vi "HEWH RLT PRAT.vi"() -> ()   [LabVIEW 2016] (continued)
        n823 = call "HEWH Gather Test Data.vi"("MW100"=w1875, "Core HEWH Data Station A"=w1870, "GEA2?"="GEA2_A?", "Yokogawa WT210"=w1863, "error in (no error)"=w1876, "Laurel IP Address"=w1853, "Draw Count"=w1852, "Use Emerson 5700?"=w1847) -> ("Core HEWH Data Station A"=w1854:T12, "MW100 Full Data"=w1868:string[][], "error out"=w1869:errorcluster)  [unwired: 6 in, 3 out]
        n824 = Unbundle By Name(w1854) -> ("LV Program"=w1860:T24)
        n825 = local read "Draw Station"() -> (w1864:string)
        n826 = call "HEWH RLT Selected MW100 TCs.vi"("Collect Power Data"="DAQ for A", "Show Flow Data"="Show Stand Override Flow Data A", "Station ID"=w1851, "Current Drawing Station"=w1864, "Error In"=w1869, "Station A Channels, MW100"=w1866, "MW100 Full Data"=w1868, "LV Program"=w1860) -> ("Error Out"=w1862:errorcluster, "TC Data"=w1857:string[][], "RMS Current (Amps)"=w1865:dbl, "Data (Label,Data)"=w1867:string[][])
        n827 = Build Array (concatenate)(w1880, w1867) -> (w1879:string[][])
        n828 = local read "Test CompleteA"() -> (w1848:bool)
        n829 = call "HEWH Tank Display.vi"("TC Data"=w1857, "LV Program"=w1860, "Min Temp (°F)"=50.0, "Max Temp (°F)"=140.0, "error in"=w1862, "DAQ for A"="DAQ for A", "Core HEWH Data Station A"=w1854, "Station ID"=w1851) -> ("Tank Display - Station A"=→"Tank Display - Station A":T33, "error out"=w1861:errorcluster)  [unwired: 6 in]
        n830 = Bundle By Name(cluster=w1878, "Core HEWH Data Input A"=w1854, "A Data Array"=w1879, "Core HEWH Data Input A.Test Complete"=w1848) -> (w1881:T80)
        n831 = case shown="\"HEWH\"" w1860 {
          tunnel: w1865 -> [_ w1884 w1885]
          frame Default {
          }
          frame "PRAT" {
            "Current (A)" <- w1884
          }
          frame "HEWH" {
            n832 = local write "Current (A)"(w1885) -> ()
          }
        }
        n833 = call <vilib>:"Add State(s) to Queue__jki_lib_state_machine.vi"("State(s) in (\"\")"=w1883) -> ("States Out"=w1882:string)  [unwired: 14 in]
        n834 = call "UTILITY Release Semaphore.vi"("error in (no error)"=w1861, "Refnum in"=w1877) -> ("error out"=w1872:errorcluster)  [unwired: 9 in]
      }
      frame "Data: Get MW100 (Station B)" {
        w1890 = "B" ("Prat Station")
        n835 = Unbundle By Name(w1919) -> ("B Data Array"=w1909:string[][], "Test Fixture Hardware"=w1912:T47, "Core HEWH Data Input B"=w1911:T12, "Test Fixture Hardware.Power.Yokogawa.WT210.Power VISA Yokogawa WT210"=w1902:refnum<visa-resource-name>, "RLT Station Channels.MW100.Station B Channels, MW100"=w1905:string[][])
        n836 = Unbundle By Name(w1912) -> ("Flow Rates.Laurel Hot IP Address"=w1892:string, "Analog Data.Yokogawa.MW100"=w1916:refnum<visa-resource-name>)
        n837 = property on="Cycle Count Display" class="DigNum (strict)"() -> ("Value"=w1891:i32)  [unwired: 2 in, 2 out]
        n838 = local read "Use Emerson 5700"() -> (w1886:bool)
        n839 = call "UTILITY Aquire Semaphore.vi"("error in (no error)"=w1915, "Refnum in"=w1914) -> ("error out"=w1917:errorcluster, "Refnum out"=w1918:T56)  [unwired: 7 in, 1 out]
        n840 = call "HEWH Gather Test Data.vi"("MW100"=w1916, "Core HEWH Data Station A"=w1911, "GEA2?"="GEA2_B?", "Yokogawa WT210"=w1902, "error in (no error)"=w1917, "Laurel IP Address"=w1892, "Draw Count"=w1891, "Use Emerson 5700?"=w1886) -> ("Core HEWH Data Station A"=w1893:T12, "MW100 Full Data"=w1908:string[][], "error out"=w1906:errorcluster)  [unwired: 6 in, 3 out]
        n841 = local read "Draw Station"() -> (w1903:string)
        n842 = Unbundle By Name(w1893) -> ("LV Program"=w1898:T24)
        n843 = call "HEWH RLT Selected MW100 TCs.vi"("Collect Power Data"="DAQ for B", "Show Flow Data"="Show Stand Override Flow Data B", "Station ID"=w1890, "Current Drawing Station"=w1903, "Error In"=w1906, "Station A Channels, MW100"=w1905, "MW100 Full Data"=w1908, "LV Program"=w1898) -> ("Error Out"=w1901:errorcluster, "TC Data"=w1899:string[][], "RMS Current (Amps)"=w1904:dbl, "Data (Label,Data)"=w1907:string[][])
        n844 = Build Array (concatenate)(w1909, w1907) -> (w1910:string[][])
        n845 = call "HEWH Tank Display.vi"("TC Data"=w1899, "LV Program"=w1898, "Min Temp (°F)"=50.0, "Max Temp (°F)"=140.0, "error in"=w1901, "DAQ for A"="DAQ for B", "Core HEWH Data Station A"=w1893, "Station ID"=w1890) -> ("Tank Display - Station A"=→"Tank Display - Station B":T33, "error out"=w1900:errorcluster)  [unwired: 6 in]
        n846 = local read "Test CompleteB"() -> (w1887:bool)
        n847 = Bundle By Name(cluster=w1919, "Core HEWH Data Input B"=w1893, "B Data Array"=w1910, "Core HEWH Data Input B.Test Complete"=w1887) -> (w1920:T80)
        n848 = case shown="\"HEWH\"" w1898 {
          tunnel: w1904 -> [_ w1923 w1924]
          frame Default {
          }
          frame "PRAT" {
            "Current (B)" <- w1923
          }
          frame "HEWH" {
            n849 = local write "Current (B)"(w1924) -> ()
          }
        }
        n850 = call "UTILITY Release Semaphore.vi"("error in (no error)"=w1900, "Refnum in"=w1918) -> ("error out"=w1913:errorcluster)  [unwired: 9 in]
        n851 = call <vilib>:"Add State(s) to Queue__jki_lib_state_machine.vi"("State(s) in (\"\")"=w1922) -> ("States Out"=w1921:string)  [unwired: 14 in]
      }
      frame "Data: Get MW100 (Station C)" {
        w1929 = "C" ("Prat Station")
        n852 = Unbundle By Name(w1958) -> ("C Data Array"=w1948:string[][], "Test Fixture Hardware"=w1951:T47, "Core HEWH Data Input C"=w1950:T12, "Test Fixture Hardware.Power.Yokogawa.WT210.Power VISA Yokogawa WT210"=w1941:refnum<visa-resource-name>, "RLT Station Channels.MW100.Station C Channels, MW100"=w1944:string[][])
        n853 = property on="Cycle Count Display" class="DigNum (strict)"() -> ("Value"=w1930:i32)  [unwired: 2 in, 2 out]
        n854 = local read "Use Emerson 5700"() -> (w1925:bool)
        n855 = Unbundle By Name(w1951) -> ("Flow Rates.Laurel Hot IP Address"=w1931:string, "Analog Data.Yokogawa.MW100"=w1955:refnum<visa-resource-name>)
        n856 = call "UTILITY Aquire Semaphore.vi"("error in (no error)"=w1954, "Refnum in"=w1953) -> ("error out"=w1956:errorcluster, "Refnum out"=w1957:T56)  [unwired: 7 in, 1 out]
        n857 = call "HEWH Gather Test Data.vi"("MW100"=w1955, "Core HEWH Data Station A"=w1950, "GEA2?"="GEA2_C?", "Yokogawa WT210"=w1941, "error in (no error)"=w1956, "Laurel IP Address"=w1931, "Draw Count"=w1930, "Use Emerson 5700?"=w1925) -> ("Core HEWH Data Station A"=w1932:T12, "MW100 Full Data"=w1946:string[][], "error out"=w1947:errorcluster)  [unwired: 6 in, 3 out]
        n858 = local read "Draw Station"() -> (w1942:string)
        n859 = Unbundle By Name(w1932) -> ("LV Program"=w1935:T24)
        n860 = call "HEWH RLT Selected MW100 TCs.vi"("Collect Power Data"="DAQ for C", "Show Flow Data"="Show Stand Override Flow Data C", "Station ID"=w1929, "Current Drawing Station"=w1942, "Error In"=w1947, "Station A Channels, MW100"=w1944, "MW100 Full Data"=w1946, "LV Program"=w1935) -> ("Error Out"=w1939:errorcluster, "TC Data"=w1940:string[][], "RMS Current (Amps)"=w1943:dbl, "Data (Label,Data)"=w1945:string[][])
        n861 = Build Array (concatenate)(w1948, w1945) -> (w1949:string[][])
        n862 = local read "Test CompleteC"() -> (w1926:bool)
        n863 = call "HEWH Tank Display.vi"("TC Data"=w1940, "LV Program"=w1935, "Min Temp (°F)"=50.0, "Max Temp (°F)"=140.0, "error in"=w1939, "DAQ for A"="DAQ for C", "Core HEWH Data Station A"=w1932, "Station ID"=w1929) -> ("Tank Display - Station A"=→"Tank Display - Station C":T33, "error out"=w1938:errorcluster)  [unwired: 6 in]
        n864 = Bundle By Name(cluster=w1958, "Core HEWH Data Input C"=w1932, "C Data Array"=w1949, "Core HEWH Data Input C.Test Complete"=w1926) -> (w1959:T80)
        n865 = case shown="\"HEWH\"" w1935 {
          tunnel: w1943 -> [_ w1962 w1963]
          frame Default {
          }
          frame "PRAT" {
            "Current (C)" <- w1962
          }
          frame "HEWH" {
            n866 = local write "Current (C)"(w1963) -> ()
          }
        }
        n867 = call "UTILITY Release Semaphore.vi"("error in (no error)"=w1938, "Refnum in"=w1957) -> ("error out"=w1952:errorcluster)  [unwired: 9 in]
        n868 = call <vilib>:"Add State(s) to Queue__jki_lib_state_machine.vi"("State(s) in (\"\")"=w1961) -> ("States Out"=w1960:string)  [unwired: 14 in]
      }
      frame "Data: Get MW100 (Station D)" {
        w1968 = "D" ("Prat Station")
        n869 = Unbundle By Name(w1997) -> ("D Data Array"=w1987:string[][], "Test Fixture Hardware"=w1990:T47, "Core HEWH Data Input D"=w1989:T12, "Test Fixture Hardware.Power.Yokogawa.WT210.Power VISA Yokogawa WT210"=w1980:refnum<visa-resource-name>, "RLT Station Channels.MW100.Station D Channels, MW100"=w1986:string[][])
        n870 = Unbundle By Name(w1990) -> ("Flow Rates.Laurel Hot IP Address"=w1970:string, "Analog Data.Yokogawa.MW100"=w1994:refnum<visa-resource-name>)
        n871 = property on="Cycle Count Display" class="DigNum (strict)"() -> ("Value"=w1969:i32)  [unwired: 2 in, 2 out]
        n872 = local read "Use Emerson 5700"() -> (w1964:bool)
        n873 = call "UTILITY Aquire Semaphore.vi"("error in (no error)"=w1993, "Refnum in"=w1992) -> ("error out"=w1995:errorcluster, "Refnum out"=w1996:T56)  [unwired: 7 in, 1 out]
        n874 = call "HEWH Gather Test Data.vi"("MW100"=w1994, "Core HEWH Data Station A"=w1989, "GEA2?"="GEA2_D?", "Yokogawa WT210"=w1980, "error in (no error)"=w1995, "Laurel IP Address"=w1970, "Draw Count"=w1969, "Use Emerson 5700?"=w1964) -> ("Core HEWH Data Station A"=w1971:T12, "MW100 Full Data"=w1984:string[][], "error out"=w1985:errorcluster)  [unwired: 6 in, 3 out]
        n875 = local read "Draw Station"() -> (w1981:string)
        n876 = Unbundle By Name(w1971) -> ("LV Program"=w1976:T24)
        n877 = call "HEWH RLT Selected MW100 TCs.vi"("Collect Power Data"="DAQ for D", "Show Flow Data"="Show Stand Override Flow Data D", "Station ID"=w1968, "Current Drawing Station"=w1981, "Error In"=w1985, "Station A Channels, MW100"=w1986, "MW100 Full Data"=w1984, "LV Program"=w1976) -> ("Error Out"=w1979:errorcluster, "TC Data"=w1977:string[][], "RMS Current (Amps)"=w1982:dbl, "Data (Label,Data)"=w1983:string[][])
        n878 = local read "Test CompleteD"() -> (w1965:bool)
        n879 = Build Array (concatenate)(w1987, w1983) -> (w1988:string[][])
        n880 = call "HEWH Tank Display.vi"("TC Data"=w1977, "LV Program"=w1976, "Min Temp (°F)"=50.0, "Max Temp (°F)"=140.0, "error in"=w1979, "DAQ for A"="DAQ for D", "Core HEWH Data Station A"=w1971, "Station ID"=w1968) -> ("Tank Display - Station A"=→"Tank Display - Station D":T33, "error out"=w1978:errorcluster)  [unwired: 6 in]
        n881 = Bundle By Name(cluster=w1997, "D Data Array"=w1988, "Core HEWH Data Input D"=w1971, "Core HEWH Data Input D.Test Complete"=w1965) -> (w1998:T80)
        n882 = case shown="\"HEWH\"" w1976 {
          tunnel: w1982 -> [_ w2001 w2002]
          frame Default {
          }
          frame "PRAT" {
            "Current (D)" <- w2001
          }
          frame "HEWH" {
            n883 = local write "Current (D)"(w2002) -> ()
          }
        }
        n884 = call "UTILITY Release Semaphore.vi"("error in (no error)"=w1978, "Refnum in"=w1996) -> ("error out"=w1991:errorcluster)  [unwired: 9 in]
        n885 = call <vilib>:"Add State(s) to Queue__jki_lib_state_machine.vi"("State(s) in (\"\")"=w2000) -> ("States Out"=w1999:string)  [unwired: 14 in]
      }
      frame "Data: Get GEA2 A" {
        # "If no GEA...you still need to \nfill in the elements into data \narray"
        # "Get the Bus Data. This is data from the actual unit"
        n886 = Unbundle By Name(w2025) -> ("GEA2 Reference Out"=w2024:refnum<k24>, "GEA2 Event Registration"=w2023:refnum<event-registration>)
        n887 = Unbundle By Name(w2031) -> ("A Data Array"=w2036:string[][], "Core HEWH Data Input A.HEWH Specific DAQ.Power State"=w2013:T22, "Core HEWH Data Input A.LV Program"=w2027:T24)
        n888 = local read "Software Version A"() -> (w2010:string)
        n889 = local read "Get Gas Data"() -> (w2006:bool)
        n890 = local read "FMA1600A Gas Data"() -> (w2005:T45)
        n891 = local read "GEA2_A?"() -> (w2003:bool)
        n892 = call "GEA2 HEWH Appliance Data.vi"(".NET Refnum in"=w2024, "LV Program"=w2027, "GEA2 Event Registration In"=w2023, "Disable Electronic Mixing Valve (EMV) List"="ERD A", "Disable Classic GEA2"=FALSE, "error in (no error)"=w2022, "#ERDs per message"="#ERDs per message", "GEA2?"=w2003, "Disable ERD A"="Disable ERD A", "Retry Count"="Retry Count") -> ("Converted Data Out"=w2015:T81, "HEWH Appliance Data ERD"=w2009:string[][], "error out"=w2012:errorcluster)  [unwired: 3 in, 4 out]
        n893 = call "HEWH Build String Diagnostics Data.vi"("Converted Data Out"=w2015, "GEA2"=w2003, "Pilot (SLPM)"="Pilot (SLPM)", "Power State Event Leads"=w2013, "Get Gas Data"=w2006, "HEWH Appliance Data ERD"=w2009, "Error In"=w2012, "Software Version A"=w2010, "FMA1600A Gas Data"=w2005) -> ("GEA Information Out"=w2007:T57, "Power Display"=w2014:T22, "Appliance Data"=w2008:string[][], "Error Out"=w2011:errorcluster)  [unwired: 3 in]
        "POWERA" <- w2014
        "POWERA Display" <- w2014
        n894 = Unbundle By Name(w2007) -> ("Water Heater GEA2 Data"=w2019:T61)
        n895 = call "HEWH Power Notifier.vi"("Status"=UTILITY_Notifier."Set", "Set Status"=w2014, "name (unnamed)"="PowerA") -> ()  [unwired: 7 in, 2 out]
        n896 = call <vilib>:"Add State(s) to Queue__jki_lib_state_machine.vi"("State(s) in (\"\")"=w2033) -> ("States Out"=w2034:string)  [unwired: 14 in]
        n897 = call "HEWH GEA Notifier.vi"("Status"=UTILITY_Notifier."Set", "Water Heater GEA2 Data"=w2019, "name (unnamed)"="GEA_A") -> ()  [unwired: 7 in, 2 out]
        n898 = Build Array (concatenate)(w2036, w2008) -> (w2035:string[][])
        n899 = Bundle By Name(cluster=w2031, "A Data Array"=w2035) -> (w2032:T80)
      }
      frame "Data: Get GEA2 B" {
        # "Get the Bus Data"
        n900 = Unbundle By Name(w2053) -> ("GEA2 Reference Out"=w2052:refnum<k24>, "GEA2 Event Registration"=w2051:refnum<event-registration>)
        n901 = Unbundle By Name(w2062) -> ("B Data Array"=w2067:string[][], "Core HEWH Data Input B.HEWH Specific DAQ.Power State"=w2038:T22, "Core HEWH Data Input B.LV Program"=w2055:T24)
        n902 = local read "#ERDs per message"() -> (w2054:i32)
        n903 = local read "Retry Count"() -> (w2056:i32)
        n904 = local read "Software Version B"() -> (w2042:string)
        n905 = local read "GEA2_B?"() -> (w2037:bool)
        n906 = call "GEA2 HEWH Appliance Data.vi"(".NET Refnum in"=w2052, "LV Program"=w2055, "GEA2 Event Registration In"=w2051, "Disable Electronic Mixing Valve (EMV) List"="ERD B", "Disable Classic GEA2"=FALSE, "error in (no error)"=w2057, "#ERDs per message"=w2054, "GEA2?"=w2037, "Disable ERD A"="Disable ERD B", "Retry Count"=w2056) -> ("Converted Data Out"=w2043:T81, "HEWH Appliance Data ERD"=w2044:string[][], "error out"=w2046:errorcluster)  [unwired: 3 in, 4 out]
        n907 = call "HEWH Build String Diagnostics Data.vi"("Converted Data Out"=w2043, "GEA2"=w2037, "Power State Event Leads"=w2038, "HEWH Appliance Data ERD"=w2044, "Error In"=w2046, "Software Version A"=w2042) -> ("GEA Information Out"=w2040:T57, "Power Display"=w2039:T22, "Appliance Data"=w2041:string[][], "Error Out"=w2045:errorcluster)  [unwired: 6 in]
        "POWERB" <- w2039
        "POWERB Display" <- w2039
        n908 = Unbundle By Name(w2040) -> ("Water Heater GEA2 Data"=w2048:T61)
        n909 = call "HEWH Power Notifier.vi"("Status"=UTILITY_Notifier."Set", "Set Status"=w2039, "name (unnamed)"="PowerB") -> ()  [unwired: 7 in, 2 out]
        n910 = call "HEWH GEA Notifier.vi"("Status"=UTILITY_Notifier."Set", "Water Heater GEA2 Data"=w2048, "name (unnamed)"="GEA_B") -> ()  [unwired: 7 in, 2 out]
        n911 = call <vilib>:"Add State(s) to Queue__jki_lib_state_machine.vi"("State(s) in (\"\")"=w2064) -> ("States Out"=w2065:string)  [unwired: 14 in]
        n912 = Build Array (concatenate)(w2067, w2041) -> (w2066:string[][])
        n913 = Bundle By Name(cluster=w2062, "B Data Array"=w2066) -> (w2063:T80)
      }
      frame "Data: Get GEA2 C" {
        # "Get the Bus Data"
        n914 = Unbundle By Name(w2084) -> ("GEA2 Reference Out"=w2083:refnum<k24>, "GEA2 Event Registration"=w2082:refnum<event-registration>)
        n915 = Unbundle By Name(w2093) -> ("C Data Array"=w2098:string[][], "Core HEWH Data Input C.HEWH Specific DAQ.Power State"=w2076:T22, "Core HEWH Data Input C.LV Program"=w2086:T24)
        n916 = local read "#ERDs per message"() -> (w2085:i32)
        n917 = local read "Software Version C"() -> (w2073:string)
        n918 = local read "Retry Count"() -> (w2087:i32)
        n919 = local read "GEA2_C?"() -> (w2068:bool)
        n920 = call "GEA2 HEWH Appliance Data.vi"(".NET Refnum in"=w2083, "LV Program"=w2086, "GEA2 Event Registration In"=w2082, "Disable Electronic Mixing Valve (EMV) List"="ERD C", "Disable Classic GEA2"=FALSE, "error in (no error)"=w2088, "#ERDs per message"=w2085, "GEA2?"=w2068, "Disable ERD A"="Disable ERD C", "Retry Count"=w2087) -> ("Converted Data Out"=w2075:T81, "HEWH Appliance Data ERD"=w2074:string[][], "error out"=w2077:errorcluster)  [unwired: 3 in, 4 out]
        n921 = call "HEWH Build String Diagnostics Data.vi"("Converted Data Out"=w2075, "GEA2"=w2068, "Power State Event Leads"=w2076, "HEWH Appliance Data ERD"=w2074, "Error In"=w2077, "Software Version A"=w2073) -> ("GEA Information Out"=w2071:T57, "Power Display"=w2070:T22, "Appliance Data"=w2069:string[][], "Error Out"=w2072:errorcluster)  [unwired: 6 in]
        "POWERC" <- w2070
        "POWERC Display" <- w2070
        n922 = Unbundle By Name(w2071) -> ("Water Heater GEA2 Data"=w2079:T61)
        n923 = call "HEWH Power Notifier.vi"("Status"=UTILITY_Notifier."Set", "Set Status"=w2070, "name (unnamed)"="PowerC") -> ()  [unwired: 7 in, 2 out]
        n924 = call "HEWH GEA Notifier.vi"("Status"=UTILITY_Notifier."Set", "Water Heater GEA2 Data"=w2079, "name (unnamed)"="GEA_C") -> ()  [unwired: 7 in, 2 out]
        n925 = call <vilib>:"Add State(s) to Queue__jki_lib_state_machine.vi"("State(s) in (\"\")"=w2095) -> ("States Out"=w2096:string)  [unwired: 14 in]
        n926 = Build Array (concatenate)(w2098, w2069) -> (w2097:string[][])
        n927 = Bundle By Name(cluster=w2093, "C Data Array"=w2097) -> (w2094:T80)
      }
      frame "Data: Get GEA2 D" {
        # "Get the Bus Data"
        n928 = Unbundle By Name(w2115) -> ("GEA2 Reference Out"=w2114:refnum<k24>, "GEA2 Event Registration"=w2113:refnum<event-registration>)
        n929 = Unbundle By Name(w2124) -> ("D Data Array"=w2129:string[][], "Core HEWH Data Input D.HEWH Specific DAQ.Power State"=w2102:T22, "Core HEWH Data Input D.LV Program"=w2117:T24)
        n930 = local read "#ERDs per message"() -> (w2116:i32)
        n931 = local read "Software Version D"() -> (w2101:string)
        n932 = local read "GEA2_D?"() -> (w2099:bool)
        n933 = local read "Retry Count"() -> (w2118:i32)
        n934 = call "GEA2 HEWH Appliance Data.vi"(".NET Refnum in"=w2114, "LV Program"=w2117, "GEA2 Event Registration In"=w2113, "Disable Electronic Mixing Valve (EMV) List"="ERD D", "Disable Classic GEA2"=FALSE, "error in (no error)"=w2119, "#ERDs per message"=w2116, "GEA2?"=w2099, "Disable ERD A"="Disable ERD D", "Retry Count"=w2118) -> ("Converted Data Out"=w2106:T81, "HEWH Appliance Data ERD"=w2100:string[][], "error out"=w2108:errorcluster)  [unwired: 3 in, 4 out]
        n935 = call "HEWH Build String Diagnostics Data.vi"("Converted Data Out"=w2106, "GEA2"=w2099, "Power State Event Leads"=w2102, "HEWH Appliance Data ERD"=w2100, "Error In"=w2108, "Software Version A"=w2101) -> ("GEA Information Out"=w2105:T57, "Power Display"=w2104:T22, "Appliance Data"=w2103:string[][], "Error Out"=w2107:errorcluster)  [unwired: 6 in]
        "POWERD" <- w2104
        "POWERD Display" <- w2104
        n936 = Unbundle By Name(w2105) -> ("Water Heater GEA2 Data"=w2110:T61)
        n937 = call "HEWH Power Notifier.vi"("Status"=UTILITY_Notifier."Set", "Set Status"=w2104, "name (unnamed)"="PowerD") -> ()  [unwired: 7 in, 2 out]
        n938 = call "HEWH GEA Notifier.vi"("Status"=UTILITY_Notifier."Set", "Water Heater GEA2 Data"=w2110, "name (unnamed)"="GEA_D") -> ()  [unwired: 7 in, 2 out]
        n939 = call <vilib>:"Add State(s) to Queue__jki_lib_state_machine.vi"("State(s) in (\"\")"=w2126) -> ("States Out"=w2127:string)  [unwired: 14 in]
        n940 = Build Array (concatenate)(w2129, w2103) -> (w2128:string[][])
        n941 = Bundle By Name(cluster=w2124, "D Data Array"=w2128) -> (w2125:T80)
      }
      frame "Data: Get Agilent" {
        # "Acquire Agilent Data"
        n942 = Unbundle By Name(w2139) -> ("RLT Station Channels"=w2134:T46, "Test Fixture Hardware"=w2146:T47, "Test Fixture Hardware.Analog Data.Agilent.TC Channels-List"=w2145:string, "A Data Array"=w2144:string[][], "B Data Array"=w2143:string[][], "C Data Array"=w2142:string[][], "D Data Array"=w2141:string[][])
        n943 = call <vilib>:"Add State(s) to Queue__jki_lib_state_machine.vi"("State(s) in (\"\")"=w2152) -> ("States Out"=w2151:string)  [unwired: 14 in]
        n944 = String Length(string=w2145) -> (length=w2149:i32)
        n945 = Greater Than 0?(x=w2149) -> (x > 0?=w2147:bool)
        n946 = case shown="True" w2147 {
          tunnel: w2148 -> [w2154 w2177]
          tunnel: [w2154 w2169] -> w2140
          tunnel: w2146 -> [_ w2176]
          tunnel: w2134 -> [_ w2155]
          tunnel: [w2153 w2159] -> w2133
          tunnel: [w2153 w2158] -> w2132
          tunnel: [w2153 w2157] -> w2131
          tunnel: [w2153 w2156] -> w2130
          frame False {
            w2153 = string[][] [] ("Data (Label,Data)")
          }
          frame True {
            n947 = call "HEWH Get Agilent Data.vi"("RLT Station Channels"=w2155, "error in (no error)"=w2177, "Test Fixture Hardware"=w2176) -> ("error out"=w2175:errorcluster, "Agilent Calibrated Cluster Array"=w2174:T50[])  [unwired: 6 in, 1 out]
            n948 = call "HEWH RLT Compile TCs For Station.vi"("Error In"=w2175, "Station ID"="A", "Agilent Cluster Array In"=w2174, "RLT Station Channels In"=w2155) -> ("Error Out"=w2172:errorcluster, "Agilent Cluster Array Out"=w2167:T50[], "RLT Station Channels Out"=w2168:T46, "Data (Label,Data)"=w2159:string[][])  [unwired: 4 in]
            n949 = call "HEWH RLT Compile TCs For Station.vi"("Error In"=w2172, "Station ID"="B", "Agilent Cluster Array In"=w2167, "RLT Station Channels In"=w2168) -> ("Error Out"=w2171:errorcluster, "Agilent Cluster Array Out"=w2165:T50[], "RLT Station Channels Out"=w2166:T46, "Data (Label,Data)"=w2158:string[][])  [unwired: 4 in]
            n950 = call "HEWH RLT Compile TCs For Station.vi"("Error In"=w2171, "Station ID"="C", "Agilent Cluster Array In"=w2165, "RLT Station Channels In"=w2166) -> ("Error Out"=w2170:errorcluster, "Agilent Cluster Array Out"=w2163:T50[], "RLT Station Channels Out"=w2164:T46, "Data (Label,Data)"=w2157:string[][])  [unwired: 4 in]
            n951 = call "HEWH RLT Compile TCs For Station.vi"("Error In"=w2170, "Station ID"="D", "Agilent Cluster Array In"=w2163, "RLT Station Channels In"=w2164) -> ("Error Out"=w2169:errorcluster, "Data (Label,Data)"=w2156:string[][])  [unwired: 4 in, 2 out]
          }
        }
        n952 = Build Array (concatenate)(w2144, w2133) -> (w2138:string[][])
        n953 = Build Array (concatenate)(w2143, w2132) -> (w2137:string[][])
        n954 = Build Array (concatenate)(w2142, w2131) -> (w2136:string[][])
        n955 = Build Array (concatenate)(w2141, w2130) -> (w2135:string[][])
        n956 = Bundle By Name(cluster=w2139, "A Data Array"=w2138, "B Data Array"=w2137, "C Data Array"=w2136, "D Data Array"=w2135) -> (w2150:T80)
      }
      frame "Get Temp and Humidity" {
        # "Acquire Temp/Humidity Data"
        n957 = Unbundle By Name(w2190) -> ("Test Fixture Hardware.ITHX-Temp Humidity.IP Address 1"=w2185:string, "Test Fixture Hardware.ITHX-Temp Humidity.Remote Port"=w2184:u16, "A Data Array"=w2194:string[][], "B Data Array"=w2193:string[][], "C Data Array"=w2192:string[][], "D Data Array"=w2191:string[][], "Core HEWH Data Input A.LV Program"=w2180:T24)
        n958 = call <vilib>:"Add State(s) to Queue__jki_lib_state_machine.vi"("State(s) in (\"\")"=w2197) -> ("States Out"=w2196:string)  [unwired: 14 in]
        n959 = call "Newport ITX-D3N.vi"("Disable Filter?"=TRUE, "Device Number (Display In Header)"="1", "error in (no error)"=w2183, "Remote Port"=w2184, "Machine"=w2185) -> ("error out"=w2182:errorcluster, "Newport ITX Data"=w2181:string[][])  [unwired: 3 in, 2 out]
        n960 = case shown="\"HEWH\", Default" w2180 {
          tunnel: w2194 -> [w2198 w2212]
          tunnel: w2193 -> [w2202 w2211]
          tunnel: w2192 -> [w2201 w2210]
          tunnel: w2191 -> [w2200 w2209]
          tunnel: [w2203 w2208] -> w2189
          tunnel: [w2202 w2207] -> w2188
          tunnel: [w2201 w2206] -> w2187
          tunnel: [w2200 w2205] -> w2186
          tunnel: w2181 -> [w2199 w2204]
          frame "HEWH", Default {
            n961 = Build Array (concatenate)(w2198, w2199) -> (w2203:string[][])
          }
          frame "PRAT", "HEWH RLT" {
            n962 = Build Array (concatenate)(w2212, w2204) -> (w2208:string[][])
            n963 = Build Array (concatenate)(w2211, w2204) -> (w2207:string[][])
            n964 = Build Array (concatenate)(w2210, w2204) -> (w2206:string[][])
            n965 = Build Array (concatenate)(w2209, w2204) -> (w2205:string[][])
          }
        }
        n966 = Bundle By Name(cluster=w2190, "A Data Array"=w2189, "B Data Array"=w2188, "C Data Array"=w2187, "D Data Array"=w2186) -> (w2195:T80)
      }
      frame "Get Gas Data" {
        # "Acquire Temp/Humidity Data"
        n967 = Unbundle By Name(w2240) -> ("A Data Array"=w2244:string[][], "B Data Array"=w2243:string[][], "C Data Array"=w2242:string[][], "D Data Array"=w2241:string[][], "Core HEWH Data Input A.LV Program"=w2235:T24, "Test Fixture Hardware.Gas Meter COM Ports.Gas Meter 1"=w2230:refnum<visa-resource-name>)
        n968 = call <vilib>:"Add State(s) to Queue__jki_lib_state_machine.vi"("State(s) in (\"\")"=w2247) -> ("States Out"=w2246:string)  [unwired: 14 in]
        n969 = call "FMA1600A Send Receive.vi"("Unit ID"="A", "error in (no error)"=w2233, "Gas Type"="Gas Type", "FMA1600A Commands"="FMA1600A Commands", "VISA Refnum in"=w2230) -> ("error out"=w2234:errorcluster, "Raw FMA1600A Data"=w2213:string)  [unwired: 4 in, 1 out]
        "Raw FMA1600A Data" <- w2213
        n970 = call "FMA1600A Parse Data.vi"("Error In"=w2234, "Raw FMA1600A Data"=w2213) -> ("Error Out"=w2232:errorcluster, "FMA1600A Gas Data"=w2217:T45)  [unwired: 7 in]
        "FMA1600A Gas Data" <- w2217
        n971 = Unbundle By Name(w2217) -> ("Pressure (PSIA)"=w2221:dbl, "Temperature (°F)"=w2222:dbl, "Vol. Flow (LPM)"=w2223:dbl, "Mass Flow (SLPM)"=w2224:dbl, "Gas Type"=w2229:string)
        n972 = Number To Fractional String(number=w2221) -> (F-format string=w2225:string)  [unwired: 3 in]
        n973 = Number To Fractional String(number=w2222) -> (F-format string=w2226:string)  [unwired: 3 in]
        n974 = Number To Fractional String(number=w2223) -> (F-format string=w2227:string)  [unwired: 3 in]
        n975 = Number To Fractional String(number=w2224) -> (F-format string=w2228:string)  [unwired: 3 in]
        n976 = Build Array(w2225, w2226, w2227, w2228, w2229) -> (w2220:string[])
        n977 = Build Array(string[] ["Gas Pressure (PSIA)", "Gas Temperature (°F)", "Volumetric Flow Rate (FT³)", "Mass Flow Rate (SFT³)", "Gas Type"], w2220) -> (w2218:string[][])
        n978 = Transpose 2D Array(2D array=w2218) -> (transposed array=w2216:string[][])
        n979 = case shown="\"HEWH\", Default" w2235 {
          tunnel: w2244 -> [w2249 w2257]
          tunnel: w2243 -> [w2252 w2256]
          tunnel: w2242 -> [w2251 w2255]
          tunnel: w2241 -> [w2250 w2254]
          tunnel: [w2253 w2257] -> w2239
          tunnel: [w2252 w2256] -> w2238
          tunnel: [w2251 w2255] -> w2237
          tunnel: [w2250 w2254] -> w2236
          tunnel: w2216 -> [w2248 _]
          frame "HEWH", Default {
            n980 = Build Array (concatenate)(w2249, w2248) -> (w2253:string[][])
          }
          frame "PRAT", "HEWH RLT" {
          }
        }
        n981 = Bundle By Name(cluster=w2240, "A Data Array"=w2239, "B Data Array"=w2238, "C Data Array"=w2237, "D Data Array"=w2236) -> (w2245:T80)
      }
      frame "Data: Check Errors" {
        n982 = Unbundle By Name(w2264) -> ("A Data Array"=w2268:string[][], "B Data Array"=w2267:string[][], "C Data Array"=w2266:string[][], "D Data Array"=w2265:string[][])
        n983 = call <vilib>:"Add State(s) to Queue__jki_lib_state_machine.vi"("State(s) in (\"\")"=w2270) -> ("States Out"=w2269:string)  [unwired: 14 in]
        n984 = call "HEWH RLT Error Checker.vi"("A Data Array"=w2268, "B Data Array"=w2267, "C Data Array"=w2266, "D Data Array"=w2265, "Error In"=w2263) -> ("Alarm A"=→"Alarm A":bool, "Alarm B"=→"Alarm B":bool, "Alarm C"=→"Alarm C":bool, "Alarm D"=→"Alarm D":bool, "Error Out"=w2262:errorcluster)  [unwired: 6 in]
      }
      frame "Data: Update Data Path A" {
        # "For RLT and PRAT, I create a new file each cycle. Prevents very large files"
        n985 = Unbundle By Name(w2272) -> ("Display Data (RLT).Station Label Display"=w2271:string)
        n986 = case shown="True" "New File Per CycA" {
          tunnel: w2273 -> [w2282 w2300]
          tunnel: w2277 -> [w2283 w2292]
          tunnel: [w2283 w2291] -> w2276
          tunnel: [w2280 w2289] -> w2275
          tunnel: w2271 -> [_ w2286]
          frame False {
            n987 = Bundle By Name(cluster=w2282, "File Locations A.New Summary Created"=FALSE) -> (w2280:T80)
          }
          frame True {
            # "I re-purposed this control. It now\ntriggers a header write in \"Data:\nSave\""
            # "I couldnt use a local to pass data due to UI Button"
            n988 = local read "Appliance Details A"() -> (w2285:T4)
            n989 = Unbundle By Name(w2300) -> ("Core HEWH Data Input A.LV Program"=w2284:T24, "File Locations A"=w2294:T2)
            n990 = property on="Cycle Count Display" class="DigNum (strict)"() -> ("Value"=w2287:i32)  [unwired: 2 in, 2 out]
            n991 = Unbundle By Name(w2285) -> ("Appliance Common.TR Number:"=w2298:string, "Appliance Common.Lab ID:"=w2297:string, "Appliance Common.Serial Number:"=w2296:string)
            n992 = Bundle By Name(cluster=T28 {"Appliance Details"={"FileVersionInfo"={"FileVersion"="", "ProductName"="", "InternalName"="", "CompanyName"="", "LegalCopyright"="", "FileDescription"=""}, "Dishwasher Info"={"Open Cup Weight (gm):"=0.0, "Auto Cup Weight (gm):"=0.0, "Detergent-Dish:"="", "Inlet Temperature-Dish:"="", "Cycle Mode-Dish:"="", "Unit Control-Dish:"="", "Manufacturer-Dish:"=""}, "Washer Info"={"Hot Water Temperature (Fahrenheit):"="", "Cold Water Temperature (Fahrenheit):"="", "Capacity (cu.ft):"=0.0, "Initial Cloth Weight:"=0.0, "Cloth Lot:"=0, "Model Family:"="", "Program Name:"="", "Cycle Selection:"="", "Wash Temperature:"="", "Rinse Temperature:"="", "Load Size:"=""}, "File Name Output Array"=[], "Calibration Output Array"=[], "Appliance Common"={"Engineer:"="", "Model Number:"="", "Serial Number:"="", "Comments:"="", "Station ID:"="", "Technician:"="", "TR Number:"="", "Lab ID:"="", "Voltage:"="", "Water Pressure (PSI):"="", "Test Date:"="", "Computer Name:"="", "IP Address:"="", "Ambient RH:"="", "Frequency:"="", "Build:"="", "Filename:"="", "Test Type:"="", "Load Run #:"=0, "Ambient Temperature (F):"="", "File Path:"=path "", "Cycles Per Year"=60}, "Water Heater"={"Heating Mode:"=""}, "Dryer"={"Heat Setting:"="", "Washer Water Temperature (60 ± 5°F):"=60, "Water Hardness (PPM):"=17, "Dryness Setting:"="", "Dryer Type:"="", "Exhaust:"="", "Drying Cycle:"="", "Load Type:"="", "Nominal Load Weight"="", "Dryer Initial IMC Data"={"Measured IMC (lbs)"=7.0, "Actual Initial RMC (%)"=7.0, "RMC (Desired %)"=100.0, "Bone Dry Wt(lbs)"=7.0, "Tolerance(%)"=5.0, "Actual Final RMC (%)"=0.0, "CEF (lbf/kWh)"=0.0, "Minimum Weight (lbf)"=0.0, "Average Weight (lbf)"=0.0, "Maximum Weight (lbf)"=0.0, "Measured IMC In Range?"=FALSE, "Moisture Reduction Factor"=55.5, "Field Use Factor"=1.04, "Empty Dryer Cold Weigth"=0.0, "Energy Standard"=enum."D2-Automatic Dryer", "Weight Cloth (lbs)"=0.0, "Relative Moisture Content (%)"=0.0, "Relative Moisture Content - Avg (%)"=0.0}}}, "Display Data (RLT)"={"Status Color"=0, "Serial Number Display"="", "Cycle Count Display"=0, "Station Label Display"="", "Current Run Start Time Display"=0.0, "Board ID Display"="", "RPM Display"=0, "Current Display"=0.0, "Current Path Display"=path "", "Saving Display"=FALSE, "Unit Type Display"=enum."", "Total Time On Display"=0.0, "UI Button"=FALSE}} ("Initialize.Washer In"), "Appliance Details.Appliance Common.TR Number:"=w2298, "Appliance Details.Appliance Common.Lab ID:"=w2297, "Appliance Details.Appliance Common.Serial Number:"=w2296, "Display Data (RLT).Station Label Display"=w2286, "Display Data (RLT).Cycle Count Display"=w2287) -> (w2295:T28)
            n993 = call "Save File Format All Folders.vi"("LV Program"=w2284, "error in (no error)"=w2292, "Initialize.Washer In"=w2295, "File Locations In"=w2294) -> ("error out"=w2291:errorcluster, "New File?"=w2288:bool, "File Locations Out"=w2293:T2)  [unwired: 5 in]
            n994 = Bundle By Name(cluster=w2300, "File Locations A"=w2293) -> (w2290:T80)
            n995 = Bundle By Name(cluster=w2290, "File Locations A.New Summary Created"=w2288) -> (w2289:T80)
          }
        }
        n996 = call <vilib>:"Add State(s) to Queue__jki_lib_state_machine.vi"("State(s) in (\"\")"=w2279) -> ("States Out"=w2278:string)  [unwired: 14 in]
      }
      frame "Data: Update Data Path B" {
        n997 = Unbundle By Name(w2302) -> ("Display Data (RLT).Station Label Display"=w2301:string)
        n998 = case shown="True" "New File Per CycB" {
          tunnel: w2307 -> [w2312 w2330]
          tunnel: w2306 -> [w2313 w2322]
          tunnel: [w2313 w2321] -> w2305
          tunnel: [w2311 w2319] -> w2304
          tunnel: w2301 -> [_ w2315]
          frame False {
            n999 = Bundle By Name(cluster=w2312, "File Locations B.New Summary Created"=FALSE) -> (w2311:T80)
          }
          frame True {
            # "I re-purposed this control. It now\ntriggers a header write in \"Data:\nSave\""
            # "I couldnt use a local to pass data due to UI Button"
            n1000 = local read "Appliance Details B"() -> (w2316:T4)
            n1001 = Unbundle By Name(w2330) -> ("Core HEWH Data Input B.LV Program"=w2314:T24, "File Locations B"=w2325:T2)
            n1002 = property on="Cycle Count Display" class="DigNum (strict)"() -> ("Value"=w2317:i32)  [unwired: 2 in, 2 out]
            n1003 = Unbundle By Name(w2316) -> ("Appliance Common.TR Number:"=w2328:string, "Appliance Common.Lab ID:"=w2327:string, "Appliance Common.Serial Number:"=w2326:string)
            n1004 = Bundle By Name(cluster=T28 {"Appliance Details"={"FileVersionInfo"={"FileVersion"="", "ProductName"="", "InternalName"="", "CompanyName"="", "LegalCopyright"="", "FileDescription"=""}, "Dishwasher Info"={"Open Cup Weight (gm):"=0.0, "Auto Cup Weight (gm):"=0.0, "Detergent-Dish:"="", "Inlet Temperature-Dish:"="", "Cycle Mode-Dish:"="", "Unit Control-Dish:"="", "Manufacturer-Dish:"=""}, "Washer Info"={"Hot Water Temperature (Fahrenheit):"="", "Cold Water Temperature (Fahrenheit):"="", "Capacity (cu.ft):"=0.0, "Initial Cloth Weight:"=0.0, "Cloth Lot:"=0, "Model Family:"="", "Program Name:"="", "Cycle Selection:"="", "Wash Temperature:"="", "Rinse Temperature:"="", "Load Size:"=""}, "File Name Output Array"=[], "Calibration Output Array"=[], "Appliance Common"={"Engineer:"="", "Model Number:"="", "Serial Number:"="", "Comments:"="", "Station ID:"="", "Technician:"="", "TR Number:"="", "Lab ID:"="", "Voltage:"="", "Water Pressure (PSI):"="", "Test Date:"="", "Computer Name:"="", "IP Address:"="", "Ambient RH:"="", "Frequency:"="", "Build:"="", "Filename:"="", "Test Type:"="", "Load Run #:"=0, "Ambient Temperature (F):"="", "File Path:"=path "", "Cycles Per Year"=60}, "Water Heater"={"Heating Mode:"=""}, "Dryer"={"Heat Setting:"="", "Washer Water Temperature (60 ± 5°F):"=60, "Water Hardness (PPM):"=17, "Dryness Setting:"="", "Dryer Type:"="", "Exhaust:"="", "Drying Cycle:"="", "Load Type:"="", "Nominal Load Weight"="", "Dryer Initial IMC Data"={"Measured IMC (lbs)"=7.0, "Actual Initial RMC (%)"=7.0, "RMC (Desired %)"=100.0, "Bone Dry Wt(lbs)"=7.0, "Tolerance(%)"=5.0, "Actual Final RMC (%)"=0.0, "CEF (lbf/kWh)"=0.0, "Minimum Weight (lbf)"=0.0, "Average Weight (lbf)"=0.0, "Maximum Weight (lbf)"=0.0, "Measured IMC In Range?"=FALSE, "Moisture Reduction Factor"=55.5, "Field Use Factor"=1.04, "Empty Dryer Cold Weigth"=0.0, "Energy Standard"=enum."D2-Automatic Dryer", "Weight Cloth (lbs)"=0.0, "Relative Moisture Content (%)"=0.0, "Relative Moisture Content - Avg (%)"=0.0}}}, "Display Data (RLT)"={"Status Color"=0, "Serial Number Display"="", "Cycle Count Display"=0, "Station Label Display"="", "Current Run Start Time Display"=0.0, "Board ID Display"="", "RPM Display"=0, "Current Display"=0.0, "Current Path Display"=path "", "Saving Display"=FALSE, "Unit Type Display"=enum."", "Total Time On Display"=0.0, "UI Button"=FALSE}} ("Initialize.Washer In"), "Appliance Details.Appliance Common.TR Number:"=w2328, "Appliance Details.Appliance Common.Lab ID:"=w2327, "Appliance Details.Appliance Common.Serial Number:"=w2326, "Display Data (RLT).Station Label Display"=w2315, "Display Data (RLT).Cycle Count Display"=w2317) -> (w2324:T28)
            n1005 = call "Save File Format All Folders.vi"("LV Program"=w2314, "error in (no error)"=w2322, "Initialize.Washer In"=w2324, "File Locations In"=w2325) -> ("error out"=w2321:errorcluster, "New File?"=w2318:bool, "File Locations Out"=w2323:T2)  [unwired: 5 in]
            n1006 = Bundle By Name(cluster=w2330, "File Locations B"=w2323) -> (w2320:T80)
            n1007 = Bundle By Name(cluster=w2320, "File Locations B.New Summary Created"=w2318) -> (w2319:T80)
          }
        }
        n1008 = call <vilib>:"Add State(s) to Queue__jki_lib_state_machine.vi"("State(s) in (\"\")"=w2309) -> ("States Out"=w2308:string)  [unwired: 14 in]
      }
      frame "Data: Update Data Path C" {
        n1009 = Unbundle By Name(w2332) -> ("Display Data (RLT).Station Label Display"=w2331:string)
        n1010 = case shown="True" "New File Per CycC" {
          tunnel: w2337 -> [w2342 w2360]
          tunnel: w2336 -> [w2343 w2352]
          tunnel: [w2343 w2351] -> w2335
          tunnel: [w2341 w2348] -> w2334
          tunnel: w2331 -> [_ w2346]
          frame False {
            n1011 = Bundle By Name(cluster=w2342, "File Locations C.New Summary Created"=FALSE) -> (w2341:T80)
          }
          frame True {
            # "I re-purposed this control. It now\ntriggers a header write in \"Data:\nSave\""
            # "I couldnt use a local to pass data due to UI Button"
            n1012 = local read "Appliance Details C"() -> (w2345:T4)
            n1013 = property on="Cycle Count Display" class="DigNum (strict)"() -> ("Value"=w2347:i32)  [unwired: 2 in, 2 out]
            n1014 = Unbundle By Name(w2360) -> ("Core HEWH Data Input C.LV Program"=w2344:T24, "File Locations C"=w2355:T2)
            n1015 = Unbundle By Name(w2345) -> ("Appliance Common.TR Number:"=w2358:string, "Appliance Common.Lab ID:"=w2357:string, "Appliance Common.Serial Number:"=w2356:string)
            n1016 = Bundle By Name(cluster=T28 {"Appliance Details"={"FileVersionInfo"={"FileVersion"="", "ProductName"="", "InternalName"="", "CompanyName"="", "LegalCopyright"="", "FileDescription"=""}, "Dishwasher Info"={"Open Cup Weight (gm):"=0.0, "Auto Cup Weight (gm):"=0.0, "Detergent-Dish:"="", "Inlet Temperature-Dish:"="", "Cycle Mode-Dish:"="", "Unit Control-Dish:"="", "Manufacturer-Dish:"=""}, "Washer Info"={"Hot Water Temperature (Fahrenheit):"="", "Cold Water Temperature (Fahrenheit):"="", "Capacity (cu.ft):"=0.0, "Initial Cloth Weight:"=0.0, "Cloth Lot:"=0, "Model Family:"="", "Program Name:"="", "Cycle Selection:"="", "Wash Temperature:"="", "Rinse Temperature:"="", "Load Size:"=""}, "File Name Output Array"=[], "Calibration Output Array"=[], "Appliance Common"={"Engineer:"="", "Model Number:"="", "Serial Number:"="", "Comments:"="", "Station ID:"="", "Technician:"="", "TR Number:"="", "Lab ID:"="", "Voltage:"="", "Water Pressure (PSI):"="", "Test Date:"="", "Computer Name:"="", "IP Address:"="", "Ambient RH:"="", "Frequency:"="", "Build:"="", "Filename:"="", "Test Type:"="", "Load Run #:"=0, "Ambient Temperature (F):"="", "File Path:"=path "", "Cycles Per Year"=60}, "Water Heater"={"Heating Mode:"=""}, "Dryer"={"Heat Setting:"="", "Washer Water Temperature (60 ± 5°F):"=60, "Water Hardness (PPM):"=17, "Dryness Setting:"="", "Dryer Type:"="", "Exhaust:"="", "Drying Cycle:"="", "Load Type:"="", "Nominal Load Weight"="", "Dryer Initial IMC Data"={"Measured IMC (lbs)"=7.0, "Actual Initial RMC (%)"=7.0, "RMC (Desired %)"=100.0, "Bone Dry Wt(lbs)"=7.0, "Tolerance(%)"=5.0, "Actual Final RMC (%)"=0.0, "CEF (lbf/kWh)"=0.0, "Minimum Weight (lbf)"=0.0, "Average Weight (lbf)"=0.0, "Maximum Weight (lbf)"=0.0, "Measured IMC In Range?"=FALSE, "Moisture Reduction Factor"=55.5, "Field Use Factor"=1.04, "Empty Dryer Cold Weigth"=0.0, "Energy Standard"=enum."D2-Automatic Dryer", "Weight Cloth (lbs)"=0.0, "Relative Moisture Content (%)"=0.0, "Relative Moisture Content - Avg (%)"=0.0}}}, "Display Data (RLT)"={"Status Color"=0, "Serial Number Display"="", "Cycle Count Display"=0, "Station Label Display"="", "Current Run Start Time Display"=0.0, "Board ID Display"="", "RPM Display"=0, "Current Display"=0.0, "Current Path Display"=path "", "Saving Display"=FALSE, "Unit Type Display"=enum."", "Total Time On Display"=0.0, "UI Button"=FALSE}} ("Initialize.Washer In"), "Appliance Details.Appliance Common.TR Number:"=w2358, "Appliance Details.Appliance Common.Lab ID:"=w2357, "Appliance Details.Appliance Common.Serial Number:"=w2356, "Display Data (RLT).Station Label Display"=w2346, "Display Data (RLT).Cycle Count Display"=w2347) -> (w2354:T28)
            n1017 = call "Save File Format All Folders.vi"("LV Program"=w2344, "error in (no error)"=w2352, "Initialize.Washer In"=w2354, "File Locations In"=w2355) -> ("error out"=w2351:errorcluster, "New File?"=w2350:bool, "File Locations Out"=w2353:T2)  [unwired: 5 in]
            n1018 = Bundle By Name(cluster=w2360, "File Locations C"=w2353) -> (w2349:T80)
            n1019 = Bundle By Name(cluster=w2349, "File Locations C.New Summary Created"=w2350) -> (w2348:T80)
          }
        }
        n1020 = call <vilib>:"Add State(s) to Queue__jki_lib_state_machine.vi"("State(s) in (\"\")"=w2339) -> ("States Out"=w2338:string)  [unwired: 14 in]
      }
      frame "Data: Update Data Path D" {
        n1021 = case shown="True" "New File Per CycD" {
          tunnel: w2366 -> [w2371 w2390]
          tunnel: w2365 -> [w2372 w2382]
          tunnel: [w2372 w2381] -> w2364
          tunnel: [w2370 w2378] -> w2363
          tunnel: w2361 -> [_ w2375]
          frame False {
            n1022 = Bundle By Name(cluster=w2371, "File Locations D.New Summary Created"=FALSE) -> (w2370:T80)
          }
          frame True {
            # "I re-purposed this control. It now\ntriggers a header write in \"Data:\nSave\""
            # "I couldnt use a local to pass data due to UI Button"
            n1023 = local read "Appliance Details D"() -> (w2376:T4)
            n1024 = Unbundle By Name(w2375) -> ("Display Data (RLT).Station Label Display"=w2374:string)
            n1025 = property on="Cycle Count Display" class="DigNum (strict)"() -> ("Value"=w2377:i32)  [unwired: 2 in, 2 out]
            n1026 = Unbundle By Name(w2390) -> ("Core HEWH Data Input D.LV Program"=w2373:T24, "File Locations D"=w2385:T2)
            n1027 = Unbundle By Name(w2376) -> ("Appliance Common.TR Number:"=w2388:string, "Appliance Common.Lab ID:"=w2387:string, "Appliance Common.Serial Number:"=w2386:string)
            n1028 = Bundle By Name(cluster=T28 {"Appliance Details"={"FileVersionInfo"={"FileVersion"="", "ProductName"="", "InternalName"="", "CompanyName"="", "LegalCopyright"="", "FileDescription"=""}, "Dishwasher Info"={"Open Cup Weight (gm):"=0.0, "Auto Cup Weight (gm):"=0.0, "Detergent-Dish:"="", "Inlet Temperature-Dish:"="", "Cycle Mode-Dish:"="", "Unit Control-Dish:"="", "Manufacturer-Dish:"=""}, "Washer Info"={"Hot Water Temperature (Fahrenheit):"="", "Cold Water Temperature (Fahrenheit):"="", "Capacity (cu.ft):"=0.0, "Initial Cloth Weight:"=0.0, "Cloth Lot:"=0, "Model Family:"="", "Program Name:"="", "Cycle Selection:"="", "Wash Temperature:"="", "Rinse Temperature:"="", "Load Size:"=""}, "File Name Output Array"=[], "Calibration Output Array"=[], "Appliance Common"={"Engineer:"="", "Model Number:"="", "Serial Number:"="", "Comments:"="", "Station ID:"="", "Technician:"="", "TR Number:"="", "Lab ID:"="", "Voltage:"="", "Water Pressure (PSI):"="", "Test Date:"="", "Computer Name:"="", "IP Address:"="", "Ambient RH:"="", "Frequency:"="", "Build:"="", "Filename:"="", "Test Type:"="", "Load Run #:"=0, "Ambient Temperature (F):"="", "File Path:"=path "", "Cycles Per Year"=60}, "Water Heater"={"Heating Mode:"=""}, "Dryer"={"Heat Setting:"="", "Washer Water Temperature (60 ± 5°F):"=60, "Water Hardness (PPM):"=17, "Dryness Setting:"="", "Dryer Type:"="", "Exhaust:"="", "Drying Cycle:"="", "Load Type:"="", "Nominal Load Weight"="", "Dryer Initial IMC Data"={"Measured IMC (lbs)"=7.0, "Actual Initial RMC (%)"=7.0, "RMC (Desired %)"=100.0, "Bone Dry Wt(lbs)"=7.0, "Tolerance(%)"=5.0, "Actual Final RMC (%)"=0.0, "CEF (lbf/kWh)"=0.0, "Minimum Weight (lbf)"=0.0, "Average Weight (lbf)"=0.0, "Maximum Weight (lbf)"=0.0, "Measured IMC In Range?"=FALSE, "Moisture Reduction Factor"=55.5, "Field Use Factor"=1.04, "Empty Dryer Cold Weigth"=0.0, "Energy Standard"=enum."D2-Automatic Dryer", "Weight Cloth (lbs)"=0.0, "Relative Moisture Content (%)"=0.0, "Relative Moisture Content - Avg (%)"=0.0}}}, "Display Data (RLT)"={"Status Color"=0, "Serial Number Display"="", "Cycle Count Display"=0, "Station Label Display"="", "Current Run Start Time Display"=0.0, "Board ID Display"="", "RPM Display"=0, "Current Display"=0.0, "Current Path Display"=path "", "Saving Display"=FALSE, "Unit Type Display"=enum."", "Total Time On Display"=0.0, "UI Button"=FALSE}} ("Initialize.Washer In"), "Appliance Details.Appliance Common.TR Number:"=w2388, "Appliance Details.Appliance Common.Lab ID:"=w2387, "Appliance Details.Appliance Common.Serial Number:"=w2386, "Display Data (RLT).Station Label Display"=w2374, "Display Data (RLT).Cycle Count Display"=w2377) -> (w2384:T28)
            n1029 = call "Save File Format All Folders.vi"("LV Program"=w2373, "error in (no error)"=w2382, "Initialize.Washer In"=w2384, "File Locations In"=w2385) -> ("error out"=w2381:errorcluster, "New File?"=w2380:bool, "File Locations Out"=w2383:T2)  [unwired: 5 in]
            n1030 = Bundle By Name(cluster=w2390, "File Locations D"=w2383) -> (w2379:T80)
            n1031 = Bundle By Name(cluster=w2379, "File Locations D.New Summary Created"=w2380) -> (w2378:T80)
          }
        }
        n1032 = call <vilib>:"Add State(s) to Queue__jki_lib_state_machine.vi"("State(s) in (\"\")"=w2368) -> ("States Out"=w2367:string)  [unwired: 14 in]
      }
      frame "Data: Update RLT Channels" {
        # "Update the RLT Station Channels Control"
        n1033 = Unbundle By Name(w2419) -> ("Core HEWH Data Input A.LV Program"=w2414:T24, "A Data Array"=w2398:string[][], "B Data Array"=w2397:string[][], "C Data Array"=w2396:string[][], "D Data Array"=w2395:string[][], "File Locations A"=w2418:T2, "File Locations B"=w2417:T2, "File Locations C"=w2416:T2, "File Locations D"=w2415:T2, "Core HEWH Data Input D"=w2403:T12, "Core HEWH Data Input C"=w2405:T12, "Core HEWH Data Input B"=w2406:T12, "Core HEWH Data Input A"=w2407:T12)
        "Station A" <- w2398
        "Station B" <- w2397
        "Station C" <- w2396
        "Station D" <- w2395
        "Station A SO Display" <- w2398
        "Station B SO Display" <- w2397
        "Station C SO Display" <- w2396
        "Station D SO Display" <- w2395
        n1034 = local read "Condition A"() -> (w2394:T1)
        n1035 = local read "Condition B"() -> (w2393:T1)
        n1036 = local read "Station A Test Sequence"() -> (w2402:T14[])
        n1037 = local read "Station B Test Sequence"() -> (w2401:T14[])
        n1038 = local read "Current Draw Parameters"() -> (w2412:T41)
        n1039 = local read "Station C Test Sequence"() -> (w2400:T14[])
        n1040 = local read "Station D Test Sequence"() -> (w2399:T14[])
        n1041 = call <vilib>:"Add State(s) to Queue__jki_lib_state_machine.vi"("State(s) in (\"\")"=w2421) -> ("States Out"=w2420:string)  [unwired: 14 in]
        n1042 = local write "File Locations A"(w2418) -> ()
        n1043 = local write "File Locations B"(w2417) -> ()
        n1044 = local write "File Locations C"(w2416) -> ()
        n1045 = local write "File Locations D"(w2415) -> ()
        n1046 = local read "Condition C"() -> (w2392:T1)
        n1047 = local read "Condition D"() -> (w2391:T1)
        n1048 = call "HEWH Update Draw Sequence Data.vi"("Core HEWH Data Input A"=w2407, "Station A Test Sequence"=w2402, "Condition B"=w2393, "Station B Test Sequence"=w2401, "Draw Parameters"=w2412, "error in (no error)"=w2413, "Core HEWH Data Input B"=w2406, "Station C Test Sequence"=w2400, "Condition A"=w2394, "Condition C"=w2392, "Core HEWH Data Input C"=w2405, "Station D Test Sequence"=w2399, "Core HEWH Data Input D"=w2403, "Condition D"=w2391) -> ("Core HEWH Data Output"=w2408:T12, "Core HEWH Data Output 2"=w2409:T12, "Core HEWH Data Output 3"=w2410:T12, "Core HEWH Data Output 4"=w2411:T12, "error out"=w2404:errorcluster)  [unwired: 1 in]
        n1049 = case shown="\"HEWH RLT\"" w2414 {
          tunnel: w2398 -> [_ w2433]
          tunnel: w2397 -> [_ w2430]
          tunnel: w2396 -> [_ w2429]
          tunnel: w2395 -> [_ w2428]
          frame Default {
          }
          frame "HEWH RLT" {
            n1050 = local read "DAQ for A"() -> (w2432:bool)
            n1051 = local read "DAQ for B"() -> (w2427:bool)
            n1052 = local read "DAQ for C"() -> (w2426:bool)
            n1053 = local read "DAQ for D"() -> (w2425:bool)
            n1054 = call "HEWH RLT Get Current.vi"("DAQ for A"=w2432, "A Data Array"=w2433) -> ("Current"=w2431:dbl)  [unwired: 8 in, 1 out]
            n1055 = call "HEWH RLT Get Current.vi"("DAQ for A"=w2427, "A Data Array"=w2430) -> ("Current"=w2424:dbl)  [unwired: 8 in, 1 out]
            n1056 = call "HEWH RLT Get Current.vi"("DAQ for A"=w2426, "A Data Array"=w2429) -> ("Current"=w2423:dbl)  [unwired: 8 in, 1 out]
            n1057 = call "HEWH RLT Get Current.vi"("DAQ for A"=w2425, "A Data Array"=w2428) -> ("Current"=w2422:dbl)  [unwired: 8 in, 1 out]
            n1058 = local write "Current (A)"(w2431) -> ()
            n1059 = local write "Current (B)"(w2424) -> ()
            n1060 = local write "Current (C)"(w2423) -> ()
            n1061 = local write "Current (D)"(w2422) -> ()
          }
        }
        n1062 = local write "Core HEWH Data Input A"(w2408) -> ()
        n1063 = local write "Core HEWH Data Input B"(w2409) -> ()
        n1064 = local write "Core HEWH Data Input C"(w2410) -> ()
        n1065 = local write "Core HEWH Data Input D"(w2411) -> ()
      }
      frame "Show Data A" {
        n1066 = Unbundle By Name(w2449) -> ("Plot Array A"=w2452:dbl[][], "A Data Array"=w2442:string[][], "File Locations A.New Summary Created"=w2443:bool, "Core HEWH Data Input A.LV Program"=w2435:T24)
        n1067 = Transpose 2D Array(2D array=w2442) -> (transposed array=w2441:string[][])
        n1068 = call <vilib>:"Add State(s) to Queue__jki_lib_state_machine.vi"("State(s) in (\"\")"=w2454) -> ("States Out"=w2453:string)  [unwired: 14 in]
        n1069 = case shown="Default" w2435 {
          tunnel: [TRUE ("Reset After 24hrs") FALSE ("Reset After 24hrs")] -> w2436
          frame Default {
          }
          frame "PRAT", "HEWH RLT" {
          }
        }
        n1070 = call "UTILITY MultiPlot.vi"("Y-Axis-2"="Y-Axis2 - Station A", "Y-Axis-1"="Y-Axis1 - Station A", "X-Axis"="X-Axis - Station A", "Save Data"=w2441, "Plot Array"=w2452) -> ("Plot Cluster"=w2450:T34)  [unwired: 5 in, 1 out]
        n1071 = call "UTILITY Create Plot Array.vi"("Save Data"=w2441, "Plot Array in"=w2452) -> ("Plot Array out"=w2440:dbl[][])  [unwired: 8 in, 1 out]
        n1072 = case shown="False" "Pause Graph" {
          tunnel: w2450 -> [w2461 _]
          tunnel: "X-Axis - Station A" -> [w2460 _]
          tunnel: "Y-Axis1 - Station A" -> [w2459 _]
          frame False {
            n1073 = property on="XY Graph - Station A" class="XYGraph (strict)"("XScale.NameLbl.Text"=w2460, "YScale.NameLbl.Text"=w2459) -> ()  [unwired: 2 in, 2 out]
            "XY Graph - Station A" <- w2461
          }
          frame True {
          }
        }
        n1074 = call "UTILITY Array Reset.vi"("Reset After 24hrs"=w2436, "Plot Array Input"=w2440) -> ("Reset Array"=w2439:bool)  [unwired: 9 in]
        n1075 = Compound Arithmetic op=OR("Clear Graph Data", w2443, w2439) -> (w2444:bool)
        n1076 = case shown="False" w2444 {
          tunnel: w2440 -> [w2457 _]
          tunnel: [w2457 dbl[][] [] ("Plot Array out")] -> w2447
          frame False {
          }
          frame True {
          }
        }
        n1077 = Bundle By Name(cluster=w2449, "Plot Array A"=w2447) -> (w2448:T80)
      }
      frame "Show Data B" {
        n1078 = Unbundle By Name(w2474) -> ("Plot Array B"=w2472:dbl[][], "B Data Array"=w2469:string[][], "File Locations B.New Summary Created"=w2471:bool, "Core HEWH Data Input B.LV Program"=w2463:T24)
        n1079 = case shown="\"PRAT\", \"HEWH RLT\"" w2463 {
          tunnel: [TRUE ("Reset After 24hrs") FALSE ("Reset After 24hrs")] -> w2462
          frame Default {
          }
          frame "PRAT", "HEWH RLT" {
          }
        }
        n1080 = Transpose 2D Array(2D array=w2469) -> (transposed array=w2468:string[][])
        n1081 = call <vilib>:"Add State(s) to Queue__jki_lib_state_machine.vi"("State(s) in (\"\")"=w2482) -> ("States Out"=w2481:string)  [unwired: 14 in]
        n1082 = call "UTILITY MultiPlot.vi"("Y-Axis-2"="Y-Axis2 - Station B", "Y-Axis-1"="Y-Axis1 - Station B", "X-Axis"="X-Axis - Station B", "Save Data"=w2468, "Plot Array"=w2472) -> ("Plot Cluster"=w2479:T34)  [unwired: 5 in, 1 out]
        n1083 = call "UTILITY Create Plot Array.vi"("Save Data"=w2468, "Plot Array in"=w2472) -> ("Plot Array out"=w2467:dbl[][])  [unwired: 8 in, 1 out]
        n1084 = case shown="False" "Pause Graph B" {
          tunnel: w2479 -> [w2489 _]
          tunnel: "X-Axis - Station B" -> [w2488 _]
          tunnel: "Y-Axis1 - Station B" -> [w2487 _]
          frame False {
            n1085 = property on="XY Graph - Station B" class="XYGraph (strict)"("XScale.NameLbl.Text"=w2488, "YScale.NameLbl.Text"=w2487) -> ()  [unwired: 2 in, 2 out]
            "XY Graph - Station B" <- w2489
          }
          frame True {
          }
        }
        n1086 = call "UTILITY Array Reset.vi"("Reset After 24hrs"=w2462, "Plot Array Input"=w2467) -> ("Reset Array"=w2466:bool)  [unwired: 9 in]
        n1087 = Compound Arithmetic op=OR("Clear Graph Data B", w2471, w2466) -> (w2475:bool)
        n1088 = case shown="False" w2475 {
          tunnel: w2467 -> [w2485 _]
          tunnel: [w2485 dbl[][] [] ("Plot Array out")] -> w2478
          frame False {
          }
          frame True {
          }
        }
        n1089 = Bundle By Name(cluster=w2474, "Plot Array B"=w2478) -> (w2473:T80)
      }
      frame "Show Data C" {
